vi "Global Plantita Parameters.vi"() -> ()   [LabVIEW 2019]
panel:
  in  "Cluster":T1
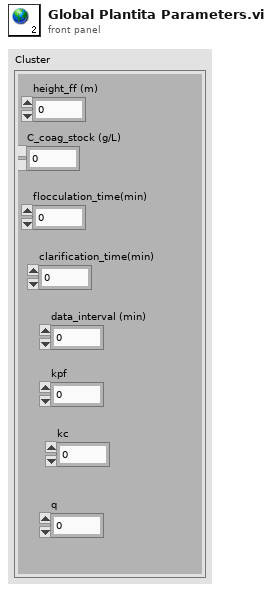
[diagram p1: front panel]
types:
  T1 = cluster{"height_ff (m)":dbl, "C_coag_stock (g/L)":dbl, "flocculation_time(min)":dbl, "clarification_time(min)":dbl, "data_interval (min)":dbl, "kpf":dbl, "kc":dbl, "q":dbl}
diagram:
